vi "1D Quadrature Integrand for Gated Decay.vi"(10 "data":variant, 11 "X":dbl[](array[numeric])) -> (0 "Error Out":errorcluster, 3 "F(X)":dbl[](array[numeric]))   [LabVIEW 2019]
doc: "This template is the starting point for creating a function that is the integrand evaluation to be passed to the Quadrature.vi."
uses:
  Gate & Decay Parameters.ctl
  Gate Type.ctl
  IRF Model.ctl
  Graphs/XY Graph/XY Plot Data.ctl
  a549e530-db8e-4861-84b1-6abd4ac2432e.vi/28aad339-045a-48ec-96ec-2fcecac66ea0.vi
  58e95aaa-8283-4ee8-aa79-031f54570487.vi/e334c8d7-bd15-48f3-9264-d19d8b21edb4.vi
  591d136b-23e2-4692-bb98-e3e8d470935c.vi/aa5492b1-e0e9-45fe-933e-8f0418e10cd1.vi
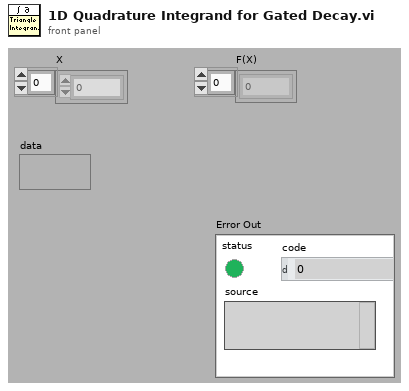
[diagram p1: front panel]
types:
  T1 = typedef "Gate & Decay Parameters.ctl" = cluster{"W":dbl, "T":dbl, "tau":dbl, "t_0":dbl, "Gate Type":T2, "t_i":dbl, "sR":dbl, "sF":dbl, "s":dbl, "Reversed Sawtooth":bool, "IRF Model":T3, "IRF Parameter 1":dbl, "User-defined Gate":T4, "Type of User-defined Function":enum32{"Gate", "IRF"}, "A":dbl}
  T2 = typedef "Gate Type.ctl" = enum16{"Square", "Finite Edge Square", "Finite Edge, Tilted Top Square", "Triangle", "Sawtooth", "User-defined"}
  T3 = typedef "IRF Model.ctl" = enum16{"Dirac", "Exponential"}
  T4 = typedef "XY Plot Data.ctl" = cluster{"X Array":dbl[], "Y Array":dbl[]}
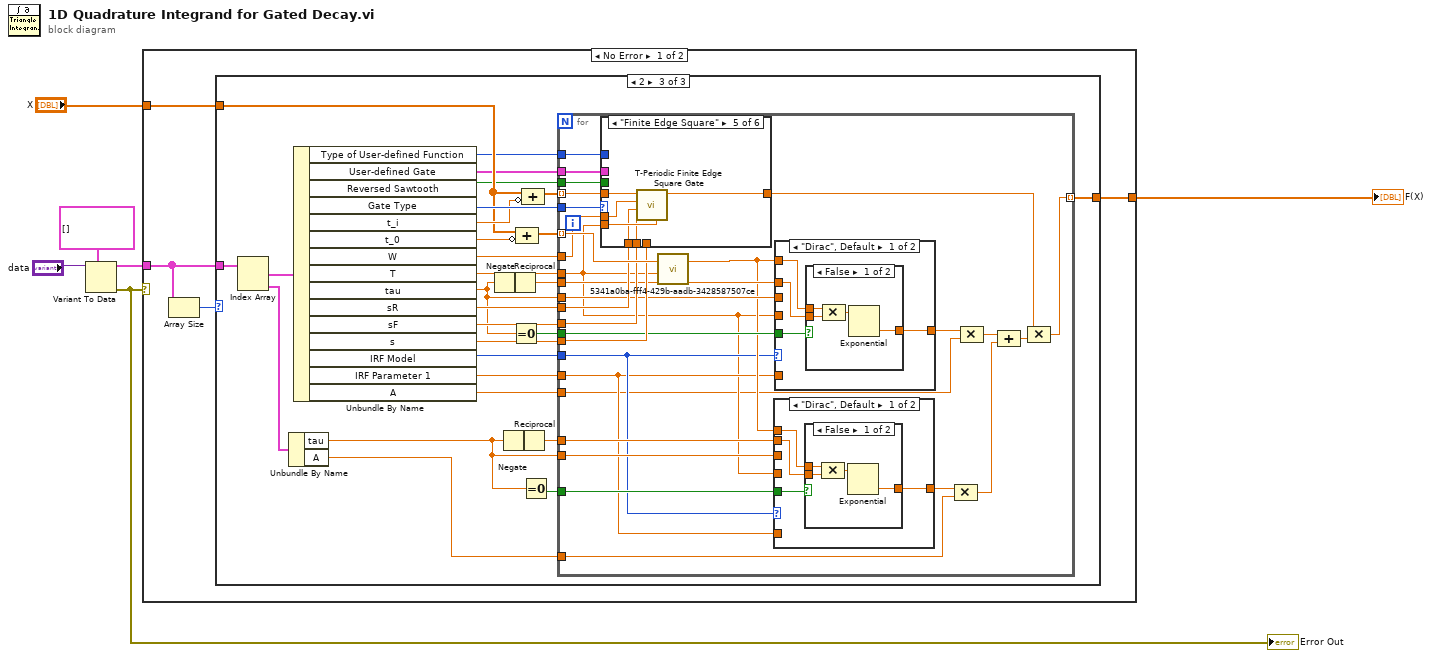
[diagram p0: block diagram]
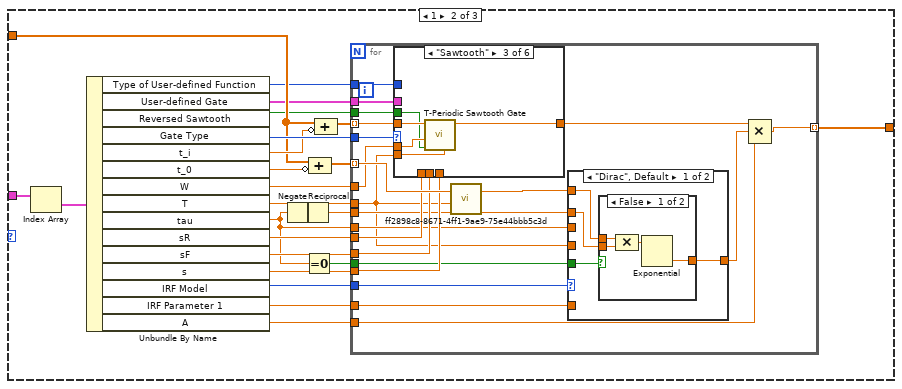
[diagram p3: hidden frame]
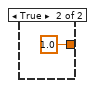
[diagram p4: hidden frame]
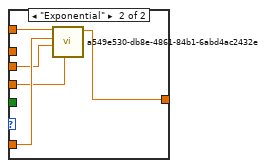
[diagram p5: hidden frame]
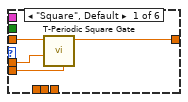
[diagram p6: hidden frame]
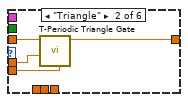
[diagram p7: hidden frame]
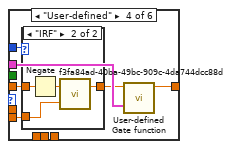
[diagram p8: hidden frame]
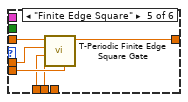
[diagram p10: hidden frame]
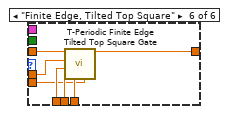
[diagram p11: hidden frame]
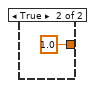
[diagram p12: hidden frame]
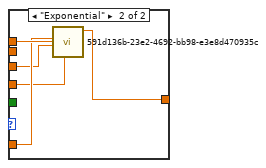
[diagram p13: hidden frame]
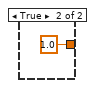
[diagram p14: hidden frame]
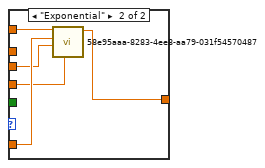
[diagram p15: hidden frame]
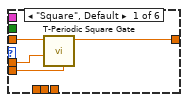
[diagram p16: hidden frame]
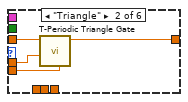
[diagram p17: hidden frame]
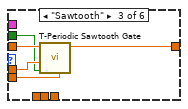
[diagram p18: hidden frame]
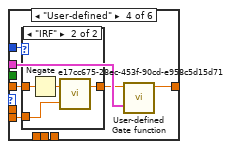
[diagram p19: hidden frame]
diagram:
  n1 = Variant To Data(type=T1[] [] ("Array"), Variant="data") -> (data=w3:T1[], error out=w2:errorcluster)  [unwired: 1 in]
  "Error Out" <- w2
  n2 = case shown="No Error" w2 {
    tunnel: "X" -> [w10 _]
    tunnel: w3 -> [w8 _]
    tunnel: [w9 _] -> w1
    frame No Error {
      n3 = Array Size(array=w8) -> (size(s)=w7:i32)
      n4 = case shown="2" w7 {
        tunnel: w10 -> [_ w28 w130]
        tunnel: [_ w14 w116] -> w9
        tunnel: w8 -> [_ w13 w115]
        frame 0, Default {
        }
        frame 1 {
          n5 = Index Array(array=w13) -> (element=w12:T1)  [unwired: 1 in]
          n6 = Unbundle By Name(w12) -> ("Type of User-defined Function"=w15:enum32{"Gate", "IRF"}, "User-defined Gate"=w18:T4, "Reversed Sawtooth"=w21:bool, "Gate Type"=w33:T2, "t_i"=w32:dbl, "t_0"=w30:dbl, "W"=w27:dbl, "T"=w34:dbl, "tau"=w17:dbl, "sR"=w24:dbl, "sF"=w23:dbl, "s"=w22:dbl, "IRF Model"=w20:T3, "IRF Parameter 1"=w19:dbl, "A"=w11:dbl)
          n7 = Negate(x=w17) -> (-x=w26:dbl)
          n8 = Reciprocal(x=w26) -> (1/x=w25:dbl)
          n9 = Equal To 0?(x=w17) -> (x = 0?=w16:bool)
          n10 = Compound Arithmetic op=ADD(w28, invert w30) -> (w29:dbl[])
          n11 = Compound Arithmetic op=ADD(w28, invert w32) -> (w31:dbl[])
          n12 = for {
            tunnel: w34 -> [w37]
            tunnel: w25 -> [w39]
            tunnel: w29 -> [w51] mode=indexing
            tunnel: w31 -> [w55] mode=indexing
            tunnel: w33 -> [w54]
            tunnel: [w53] -> w14 mode=indexing
            tunnel: w27 -> [w50]
            tunnel: w24 -> [w48]
            tunnel: w23 -> [w47]
            tunnel: w22 -> [w46]
            tunnel: w21 -> [w45]
            tunnel: w20 -> [w44]
            tunnel: w19 -> [w43]
            tunnel: w17 -> [w42]
            tunnel: w18 -> [w41]
            tunnel: w16 -> [w38]
            tunnel: w15 -> [w36]
            tunnel: w11 -> [w35]
            n13 = case shown="\"Sawtooth\"" w54 {
              tunnel: w50 -> [w72 w77 w81 _ w97 w104]
              tunnel: w55 -> [w73 w76 w82 w88 w99 w106]
              tunnel: [w71 w75 w80 w87 w98 w105] -> w52
              tunnel: w48 -> [_ _ _ _ w95 w103]
              tunnel: w47 -> [_ _ _ _ w94 w102]
              tunnel: w46 -> [_ _ _ _ _ w101]
              tunnel: w45 -> [_ _ w79 _ _ _]
              tunnel: w41 -> [_ _ _ w86 _ _]
              tunnel: w37 -> [w70 w74 w78 w85 w96 w100]
              tunnel: w36 -> [_ _ _ w83 _ _]
              frame "Square", Default {
                n14 = call "T-Periodic Square Gate.vi"("Period T"=w70, "W"=w72, "t"=w73) -> ("Square(t)"=w71:dbl)  [unwired: 8 in]
              }
              frame "Triangle" {
                n15 = call "T-Periodic Triangle Gate.vi"("Period T"=w74, "W"=w77, "t"=w76) -> ("Triangle(t)"=w75:dbl)  [unwired: 8 in]
              }
              frame "Sawtooth" {
                n16 = call "T-Periodic Sawtooth Gate.vi"("Period T"=w78, "Reversed?"=w79, "W"=w81, "t"=w82) -> ("Sawtooth(t)"=w80:dbl)  [unwired: 7 in]
              }
              frame "User-defined" {
                n17 = case shown="\"IRF\"" w83 {
                  tunnel: w88 -> [w89 w93]
                  tunnel: w85 -> [_ w91]
                  tunnel: [w89 w90] -> w84
                  frame "Gate", Default {
                  }
                  frame "IRF" {
                    n18 = Negate(x=w93) -> (-x=w92:dbl)
                    n19 = call "f3fa84ad-40ba-49bc-909c-4da744dcc88d.vi"("y"=w91, "x"=w92) -> ("x - E(x/y)y"=w90:dbl)  [unwired: 1 out]
                  }
                }
                n20 = call "User-defined Gate function.vi"("User-defined Gate"=w86, "t"=w84) -> ("User-defined Gate(t)"=w87:dbl)  [unwired: 8 in, 1 out]
              }
              frame "Finite Edge Square" {
                n21 = call "T-Periodic Finite Edge Square Gate.vi"("Period T"=w96, "s_F"=w94, "s_R"=w95, "W"=w97, "t"=w99) -> ("Finite Edge Square(t)"=w98:dbl)  [unwired: 6 in]
              }
              frame "Finite Edge, Tilted Top Square" {
                n22 = call "T-Periodic Finite Edge Tilted Top Square Gate.vi"("Period T"=w100, "slope"=w101, "s_F"=w102, "s_R"=w103, "W"=w104, "t"=w106) -> ("Finite Edge Square(t)"=w105:dbl)  [unwired: 5 in]
              }
            }
            n23 = call "ff2898c8-8671-4ff1-9ae9-75e44bbb5c3d.vi"("y"=w37, "x"=w51) -> ("x - E(x/y)y"=w40:dbl)  [unwired: 1 out]
            n24 = case shown="\"Dirac\", Default" w44 {
              tunnel: [w58 w68] -> w49
              tunnel: w40 -> [w57 w69]
              tunnel: w43 -> [_ w67]
              tunnel: w42 -> [_ w66]
              tunnel: w37 -> [_ w65]
              tunnel: w39 -> [w59 _]
              tunnel: w38 -> [w56 _]
              frame "Dirac", Default {
                n25 = case shown="False" w56 {
                  tunnel: w59 -> [w63 _]
                  tunnel: [w62 1.0] -> w58
                  tunnel: w57 -> [w61 _]
                  frame False {
                    n26 = Compound Arithmetic op=MULTIPLY(w61, w63) -> (w60:dbl)
                    n27 = Exponential(1:w60) -> (0:w62:dbl)
                  }
                  frame True {
                  }
                }
              }
              frame "Exponential" {
                n28 = call "a549e530-db8e-4861-84b1-6abd4ac2432e.vi"("Period: T"=w65, "lifetime: tau"=w66, "IRF time constant"=w67, "t"=w69) -> ("y(t)"=w68:dbl)  [unwired: 6 in, 1 out]
              }
            }
            n29 = Compound Arithmetic op=MULTIPLY(w52, w49, w35) -> (w53:dbl)
          }
        }
        frame 2 {
          n30 = Index Array(array=w115) -> (element #1=w114:T1, element #2=w113:T1)  [unwired: 2 in]
          n31 = Unbundle By Name(w113) -> ("tau"=w110:dbl, "A"=w107:dbl)
          n32 = Unbundle By Name(w114) -> ("Type of User-defined Function"=w117:enum32{"Gate", "IRF"}, "User-defined Gate"=w120:T4, "Reversed Sawtooth"=w123:bool, "Gate Type"=w135:T2, "t_i"=w134:dbl, "t_0"=w132:dbl, "W"=w129:dbl, "T"=w136:dbl, "tau"=w119:dbl, "sR"=w126:dbl, "sF"=w125:dbl, "s"=w124:dbl, "IRF Model"=w122:T3, "IRF Parameter 1"=w121:dbl, "A"=w108:dbl)
          n33 = Negate(x=w119) -> (-x=w128:dbl)
          n34 = Negate(x=w110) -> (-x=w112:dbl)
          n35 = Reciprocal(x=w128) -> (1/x=w127:dbl)
          n36 = Equal To 0?(x=w119) -> (x = 0?=w118:bool)
          n37 = Compound Arithmetic op=ADD(w130, invert w132) -> (w131:dbl[])
          n38 = Reciprocal(x=w112) -> (1/x=w111:dbl)
          n39 = Equal To 0?(x=w110) -> (x = 0?=w109:bool)
          n40 = Compound Arithmetic op=ADD(w130, invert w134) -> (w133:dbl[])
          n41 = for {
            tunnel: w136 -> [w144]
            tunnel: w127 -> [w153]
            tunnel: w131 -> [w162] mode=indexing
            tunnel: w133 -> [w165] mode=indexing
            tunnel: w135 -> [w164]
            tunnel: [w138] -> w116 mode=indexing
            tunnel: w129 -> [w161]
            tunnel: w126 -> [w159]
            tunnel: w125 -> [w158]
            tunnel: w124 -> [w157]
            tunnel: w123 -> [w156]
            tunnel: w122 -> [w146]
            tunnel: w121 -> [w145]
            tunnel: w119 -> [w155]
            tunnel: w120 -> [w154]
            tunnel: w118 -> [w152]
            tunnel: w117 -> [w151]
            tunnel: w111 -> [w149]
            tunnel: w110 -> [w148]
            tunnel: w109 -> [w147]
            tunnel: w108 -> [w143]
            tunnel: w107 -> [w141]
            n42 = case shown="\"Finite Edge Square\"" w164 {
              tunnel: w161 -> [w196 w201 w205 _ w221 w228]
              tunnel: w165 -> [w197 w200 w206 w212 w223 w230]
              tunnel: [w195 w199 w204 w211 w222 w229] -> w137
              tunnel: w159 -> [_ _ _ _ w219 w227]
              tunnel: w158 -> [_ _ _ _ w218 w226]
              tunnel: w157 -> [_ _ _ _ _ w225]
              tunnel: w156 -> [_ _ w203 _ _ _]
              tunnel: w154 -> [_ _ _ w210 _ _]
              tunnel: w144 -> [w194 w198 w202 w209 w220 w224]
              tunnel: w151 -> [_ _ _ w207 _ _]
              frame "Square", Default {
                n43 = call "T-Periodic Square Gate.vi"("Period T"=w194, "W"=w196, "t"=w197) -> ("Square(t)"=w195:dbl)  [unwired: 8 in]
              }
              frame "Triangle" {
                n44 = call "T-Periodic Triangle Gate.vi"("Period T"=w198, "W"=w201, "t"=w200) -> ("Triangle(t)"=w199:dbl)  [unwired: 8 in]
              }
              frame "Sawtooth" {
                n45 = call "T-Periodic Sawtooth Gate.vi"("Period T"=w202, "Reversed?"=w203, "W"=w205, "t"=w206) -> ("Sawtooth(t)"=w204:dbl)  [unwired: 7 in]
              }
              frame "User-defined" {
                n46 = case shown="\"IRF\"" w207 {
                  tunnel: w212 -> [w213 w217]
                  tunnel: w209 -> [_ w215]
                  tunnel: [w213 w214] -> w208
                  frame "Gate", Default {
                  }
                  frame "IRF" {
                    n47 = Negate(x=w217) -> (-x=w216:dbl)
                    n48 = call "e17cc675-28ec-453f-90cd-e958c5d15d71.vi"("y"=w215, "x"=w216) -> ("x - E(x/y)y"=w214:dbl)  [unwired: 1 out]
                  }
                }
                n49 = call "User-defined Gate function.vi"("User-defined Gate"=w210, "t"=w208) -> ("User-defined Gate(t)"=w211:dbl)  [unwired: 8 in, 1 out]
              }
              frame "Finite Edge Square" {
                n50 = call "T-Periodic Finite Edge Square Gate.vi"("Period T"=w220, "s_F"=w218, "s_R"=w219, "W"=w221, "t"=w223) -> ("Finite Edge Square(t)"=w222:dbl)  [unwired: 6 in]
              }
              frame "Finite Edge, Tilted Top Square" {
                n51 = call "T-Periodic Finite Edge Tilted Top Square Gate.vi"("Period T"=w224, "slope"=w225, "s_F"=w226, "s_R"=w227, "W"=w228, "t"=w230) -> ("Finite Edge Square(t)"=w229:dbl)  [unwired: 5 in]
              }
            }
            n52 = call "5341a0ba-fff4-429b-aadb-3428587507ce.vi"("y"=w144, "x"=w162) -> ("x - E(x/y)y"=w150:dbl)  [unwired: 1 out]
            n53 = case shown="\"Dirac\", Default" w146 {
              tunnel: [w168 w178] -> w142
              tunnel: w150 -> [w167 w179]
              tunnel: w145 -> [_ w177]
              tunnel: w148 -> [_ w176]
              tunnel: w144 -> [_ w175]
              tunnel: w149 -> [w169 _]
              tunnel: w147 -> [w166 _]
              frame "Dirac", Default {
                n54 = case shown="False" w166 {
                  tunnel: w169 -> [w173 _]
                  tunnel: [w172 1.0] -> w168
                  tunnel: w167 -> [w171 _]
                  frame False {
                    n55 = Compound Arithmetic op=MULTIPLY(w171, w173) -> (w170:dbl)
                    n56 = Exponential(1:w170) -> (0:w172:dbl)
                  }
                  frame True {
                  }
                }
              }
              frame "Exponential" {
                n57 = call "591d136b-23e2-4692-bb98-e3e8d470935c.vi"("Period: T"=w175, "lifetime: tau"=w176, "IRF time constant"=w177, "t"=w179) -> ("y(t)"=w178:dbl)  [unwired: 6 in, 1 out]
              }
            }
            n58 = case shown="\"Dirac\", Default" w146 {
              tunnel: [w182 w192] -> w160
              tunnel: w150 -> [w181 w193]
              tunnel: w145 -> [_ w191]
              tunnel: w155 -> [_ w190]
              tunnel: w144 -> [_ w189]
              tunnel: w153 -> [w183 _]
              tunnel: w152 -> [w180 _]
              frame "Dirac", Default {
                n59 = case shown="False" w180 {
                  tunnel: w183 -> [w187 _]
                  tunnel: [w186 1.0] -> w182
                  tunnel: w181 -> [w185 _]
                  frame False {
                    n60 = Compound Arithmetic op=MULTIPLY(w185, w187) -> (w184:dbl)
                    n61 = Exponential(1:w184) -> (0:w186:dbl)
                  }
                  frame True {
                  }
                }
              }
              frame "Exponential" {
                n62 = call "58e95aaa-8283-4ee8-aa79-031f54570487.vi"("Period: T"=w189, "lifetime: tau"=w190, "IRF time constant"=w191, "t"=w193) -> ("y(t)"=w192:dbl)  [unwired: 6 in, 1 out]
              }
            }
            n63 = Compound Arithmetic op=MULTIPLY(w142, w141) -> (w139:dbl)
            n64 = Compound Arithmetic op=MULTIPLY(w160, w143) -> (w163:dbl)
            n65 = Compound Arithmetic op=ADD(w163, w139) -> (w140:dbl)
            n66 = Compound Arithmetic op=MULTIPLY(w137, w140) -> (w138:dbl)
          }
        }
      }
    }
    frame Error {
    }
  }
  "F(X)" <- w1
